vi "Create.vi"(8 "error in (no error)":errorcluster, 10 "Input":string) -> (0 "error out":errorcluster, 3 "Game":refnum<class "Game.lvclass">)   [LabVIEW 2020, in "Game.lvclass"]
uses:
  Game.lvclass
  Game.lvclass/Game.ctl
  Bag/Bag.lvclass
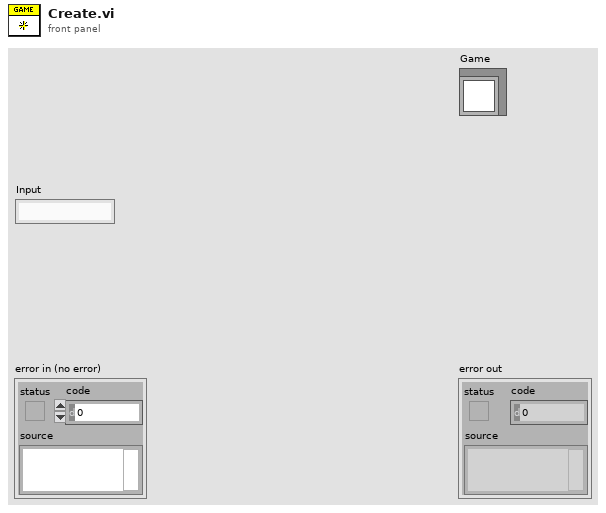
[diagram p1: front panel]
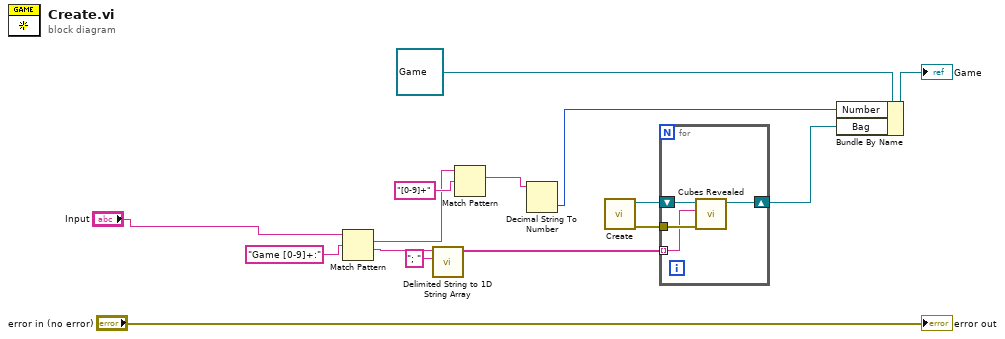
[diagram p0: block diagram]
diagram:
  n1 = Match Pattern(string="Input", regular expression="Game [0-9]+:" ("string")) -> (match substring=w3:string, after substring=w11:string)  [unwired: 1 in, 2 out]
  n2 = call <vilib>:"Delimited String to 1D String Array.vi"("delimiter"="; ", "delimited string"=w11) -> ("string array"=w5:string[])  [unwired: 9 in]
  n3 = Match Pattern(string=w3, regular expression="[0-9]+" ("string")) -> (match substring=w2:string)  [unwired: 1 in, 3 out]
  n4 = Decimal String To Number(string=w2) -> (number=w1:i32)  [unwired: 2 in, 1 out]
  n5 = call "Create.vi"() -> ("error out"=w8:errorcluster, "Bag"=w9:refnum<class "Bag.lvclass">)  [unwired: 10 in]
  n6 = for {
    tunnel: w8 -> [w18]
    shift-right: [w17] -> w6
    shift-left: w9 -> [w19]
    tunnel: w5 -> [w16] mode=indexing
    n7 = call "Cubes Revealed.vi"("error in (no error)"=w18, "Set"=w16, "Bag in"=w19) -> ("Bag out"=w17:refnum<class "Bag.lvclass">)  [unwired: 7 in, 1 out]
  }
  n8 = Bundle By Name(cluster=refnum<class "Game.lvclass"> refnum ("Game"), "Number"=w1, "Bag"=w6) -> (→"Game":refnum<class "Game.lvclass">)
  "error out" <- "error in (no error)"
